vi "CAN STP Queue Request Responce.vi"(8 "error in (no error)":errorcluster, 10 "Socket No":u16, 11 "STP Input Data":T3 {"ResponseTimeout (S)" format="%#_13g"; "+veResponseCode" format="%x"; "CMD" items=["TSW_VERSION(130)"=130, "WAIT_EVENT(132)"=132, "SEQUENCER(133)"=133, "TSW_RESET(150)"=150, "CONFIG_ECU(151)"=151, "TEST_CORE (152)"=152, "TEST_WATCHDOG (153)"=153, "TEST_MONITORING (154)"=154, "READ_MEMORY (162)"=162, "WRITE_ERASE_MEMORY (164)"=164, "COMM_EXTERNAL (190)"=190, "COMM_INTERNAL (195)"=195, "GET_ANALOG_INPUT (210)"=210, "GET_DIGITAL_INPUT (211)"=211, "GET_FREQUENCY_INPUT (212)"=212, "TEST_INPUT_STRUCTURE (214)"=214, "GENERATE_OUTPUT_SIGNAL (220)"=220, "GENERATE_SYNCHRONIZED_OUTPUT_SIGNALS (221)"=221, "eDCU_Specific (250)"=250]; "RxID" format="%.0x"; "TxID" format="%.0x"}) -> (0 "error out":errorcluster, 2 "RequestTimeout?":bool, 3 "STP Output Data":T1)   [LabVIEW 2023, in "LTT_TeststandSteptypes.lvlib"]
uses:
  LTT_TeststandSteptypes.lvlib
  HardwareAbstractionLayer_LVOOP/CAN/CAN Application Protocols/STP Protocol_class/Ctrls/STP Input Data.ctl
  HardwareAbstractionLayer_LVOOP/CAN/CAN Application Protocols/STP Protocol_class/Ctrls/STP CMD.ctl
  HardwareAbstractionLayer_LVOOP/CAN/CAN Application Protocols/STP Protocol_class/Ctrls/STP Output Data.ctl
  HardwareAbstractionLayer_LVOOP/CAN/CAN Application Protocols/STP Protocol_class/Ctrls/STP Error Cluster.ctl
  STP Engine SubVI/Control/STP Engine Tx Data.ctl
  STP Engine SubVI/Control/STP Engine Rx Data.ctl
  Control/CAN FGV State.ctl
  HardwareAbstractionLayer_LVOOP/CAN/CAN Application Protocols/STP Protocol_class/STP Protocol.lvclass
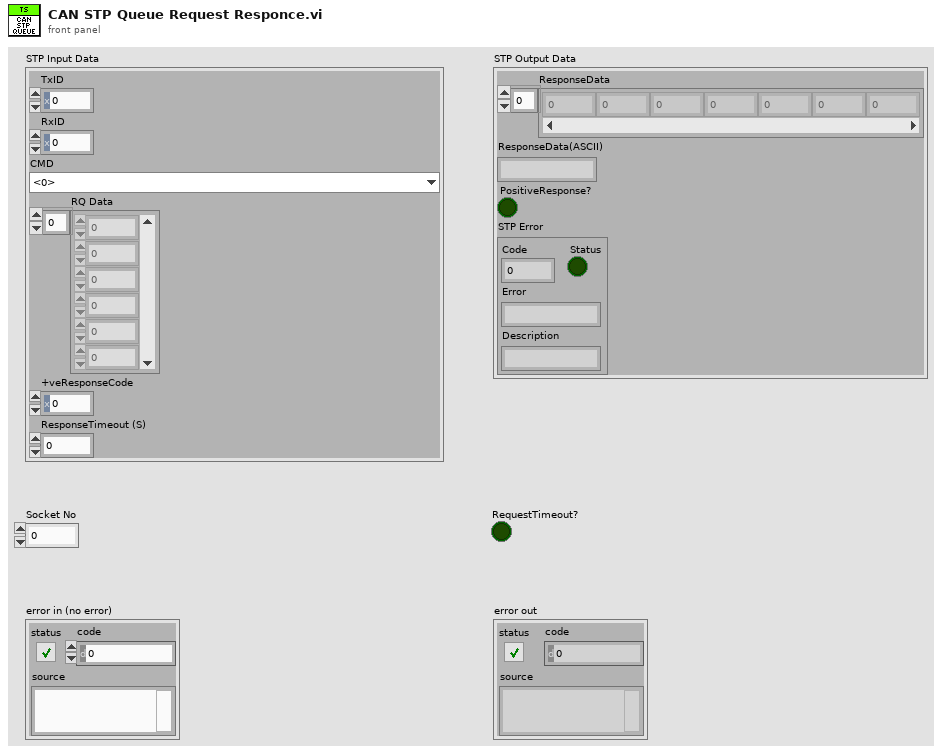
[diagram p1: front panel]
types:
  T1 = typedef "HardwareAbstractionLayer_LVOOP.lvlib/CAN Application Protocols Lib.lvlib/STP Protocol.lvclass/STP Output Data.ctl" = cluster{"ResponseData":u8[], "ResponseData(ASCII)":string, "PositiveResponse?":bool, "STP Error":T2}
  T2 = typedef "HardwareAbstractionLayer_LVOOP.lvlib/CAN Application Protocols Lib.lvlib/STP Protocol.lvclass/STP Error Cluster.ctl" = cluster{"Status":bool, "Code":u8, "Error":string, "Description":string}
  T3 = typedef "HardwareAbstractionLayer_LVOOP.lvlib/CAN Application Protocols Lib.lvlib/STP Protocol.lvclass/STP Input Data.ctl" = cluster{"TxID":u32, "RxID":u32, "CMD":T4, "RQ Data":u8[], "+veResponseCode":u8, "ResponseTimeout (S)":dbl}
  T4 = typedef "HardwareAbstractionLayer_LVOOP.lvlib/CAN Application Protocols Lib.lvlib/STP Protocol.lvclass/STP CMD.ctl" = u8
  T5 = typedef "LTT_TeststandSteptypes.lvlib/STP Engine Rx Data.ctl" = cluster{"STP Output Data":T1, "RequestTimeout?":bool}
  T6 = typedef "LTT_TeststandSteptypes.lvlib/STP Engine Tx Data.ctl" = cluster{"STP Input Data":T3, "Socket No":u16}
  T7 = typedef "LTT_TeststandSteptypes.lvlib/CAN FGV State.ctl" = enum16{"Init", "Get", "Set"}
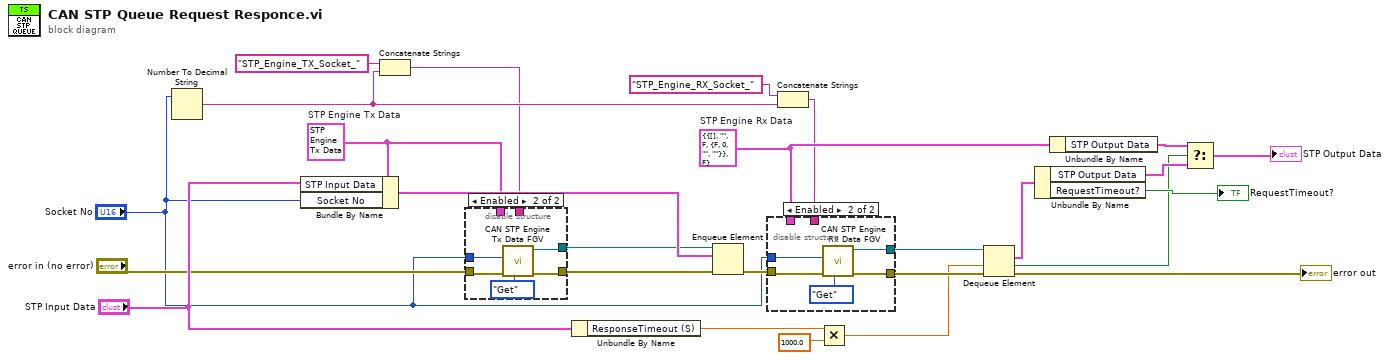
[diagram p0: block diagram]
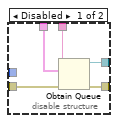
[diagram p2: hidden frame]
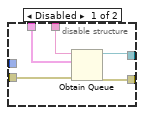
[diagram p3: hidden frame]
diagram:
  w16 = T5 {"STP Output Data"={"ResponseData"=[], "ResponseData(ASCII)"="", "PositiveResponse?"=FALSE, "STP Error"={"Status"=FALSE, "Code"=0, "Error"="", "Description"=""}}, "RequestTimeout?"=FALSE}  # STP Engine Rx Data
  w8 = T6 {"STP Input Data"={"TxID"=2042, "RxID"=2043, "CMD"=130, "RQ Data"=[], "+veResponseCode"=160, "ResponseTimeout (S)"=1.0}, "Socket No"=0}  # STP Engine Tx Data
  n1 = Number To Decimal String(number="Socket No") -> (decimal integer string=w25:string)  [unwired: 1 in]
  n2 = Bundle By Name(cluster=w8, "STP Input Data"="STP Input Data", "Socket No"="Socket No") -> (w9:T6)
  n3 = Concatenate Strings("STP_Engine_TX_Socket_", w25) -> (w6:string)
  n4 = disable-structure shown="Enabled" {
    disable-tunnel: "error in (no error)" -> [w31 w36]
    disable-tunnel: w8 -> [w30 _]
    disable-tunnel: w6 -> [w29 _]
    disable-tunnel: [w28 w35] -> w5
    disable-tunnel: [w27 w32] -> w4
    disable-tunnel: "Socket No" -> [_ w33]
    frame Disabled {
      n5 = Obtain Queue(name (unnamed)=w29, element data type=w30, error in (no error)=w31) -> (queue out=w27:refnum<queue>, error out=w28:errorcluster)  [unwired: 2 in, 1 out]
    }
    frame Enabled {
      n6 = call "CAN STP Engine Tx Data FGV.vi"("CAN FGV State"=CAN_FGV_State."Get", "error in"=w36, "Socket No"=w33) -> ("error out"=w35:errorcluster, "STP Engine Tx Data out"=w32:refnum<queue>)  [unwired: 6 in, 1 out]
    }
  }
  n7 = Unbundle By Name("STP Input Data") -> ("ResponseTimeout (S)"=w24:dbl)
  n8 = Enqueue Element(queue=w4, element=w9, error in (no error)=w5) -> (error out=w12:errorcluster)  [unwired: 1 in, 2 out]
  n9 = Concatenate Strings("STP_Engine_RX_Socket_", w25) -> (w10:string)
  n10 = disable-structure shown="Enabled" {
    disable-tunnel: w16 -> [w41 _]
    disable-tunnel: [w40 w44] -> w14
    disable-tunnel: w12 -> [w39 w45]
    disable-tunnel: w10 -> [w38 _]
    disable-tunnel: [w37 w46] -> w2
    disable-tunnel: "Socket No" -> [_ w42]
    frame Disabled {
      n11 = Obtain Queue(name (unnamed)=w38, element data type=w41, error in (no error)=w39) -> (queue out=w37:refnum<queue>, error out=w40:errorcluster)  [unwired: 2 in, 1 out]
    }
    frame Enabled {
      n12 = call "CAN STP Engine Rx Data FGV.vi"("CAN FGV State"=CAN_FGV_State."Get", "error in"=w45, "Socket No"=w42) -> ("error out"=w44:errorcluster, "STP Engine Rx Data Out"=w46:refnum<queue>)  [unwired: 7 in]
    }
  }
  n13 = Multiply(x=w24, y=1000.0) -> (x*y=w13:dbl)
  n14 = Dequeue Element(queue=w2, timeout in ms (-1)=w13, error in (no error)=w14) -> (element=w18:T5, timed out?=w15:bool, error out=→"error out":errorcluster)  [unwired: 1 out]
  n15 = Unbundle By Name(w18) -> ("STP Output Data"=w19:T1, "RequestTimeout?"=→"RequestTimeout?":bool)
  n16 = Unbundle By Name(w16) -> ("STP Output Data"=w17:T1)
  n17 = Select(t=w17, s=w15, f=w19) -> (s? t:f=→"STP Output Data":T1)
